vi "SendTCPPort.vi"(8 "error in (no error)":errorcluster, 11 "Normal Com in":refnum<class "Normal Com.lvclass">) -> (0 "error out":errorcluster, 3 "Normal Com out":refnum<class "Normal Com.lvclass">)   [LabVIEW 2023, in "Normal Com.lvclass"]
uses:
  Normal Com.lvclass
  C:/Users/santharu.subramanian/Desktop/LOA New/Documents/LV New Assignments/Sender-Receiver/Classes/Communication/Communication.lvclass
  Data/Data.lvclass
  Normal Com.lvclass/Normal Com.ctl
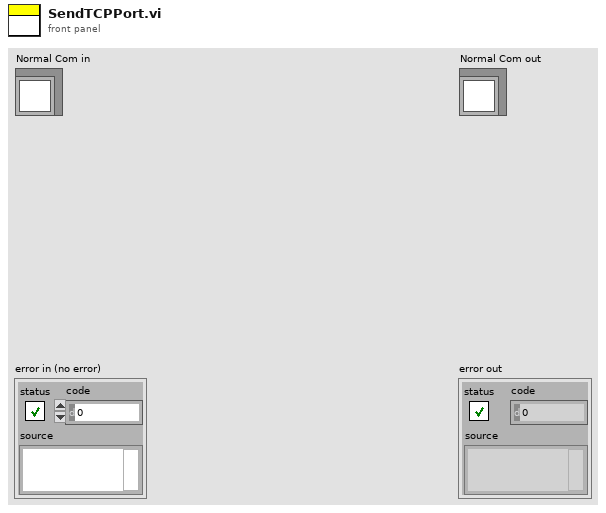
[diagram p1: front panel]
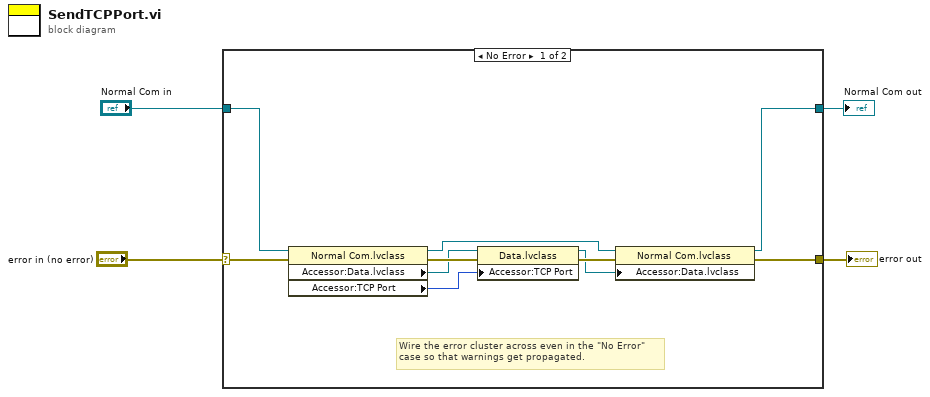
[diagram p0: block diagram]
diagram:
  n1 = case shown="No Error" "error in (no error)" {
    selector: "error in (no error)" -> [w5 w16]
    tunnel: [w6 w16] -> w3
    tunnel: [w7 w15] -> w1
    tunnel: "Normal Com in" -> [w8 w15]
    frame No Error {
      # "Wire the error cluster across even in the \"No Error\"\ncase so that warnings get propagated."
      n2 = property class="Normal Com.lvclass"(reference=w8, error in=w5) -> (reference out=w10:refnum<class "Normal Com.lvclass">, error out=w14:errorcluster, "Accessor:Data.lvclass"=w13:refnum<class "Data.lvclass">, "Accessor:TCP Port"=w12:u16)
      n3 = property class="Data.lvclass"(reference=w13, error in=w14, "Accessor:TCP Port"=w12) -> (reference out=w9:refnum<class "Data.lvclass">, error out=w11:errorcluster)
      n4 = property class="Normal Com.lvclass"(reference=w10, error in=w11, "Accessor:Data.lvclass"=w9) -> (reference out=w7:refnum<class "Normal Com.lvclass">, error out=w6:errorcluster)
    }
    frame Error {
    }
  }
  "error out" <- w3
  "Normal Com out" <- w1
